vi "SDI_CoordSpace_Test.vi"() -> ()   [LabVIEW 2014]
uses:
  <vilib>/Motion/plugins/PluginFramework/nismSDIFramework.SetFrameworkMode.multi.vi
  <vilib>/Motion/Express/_s/nimc.ex.clearFaults.clearFaults.axis.vi
  <vilib>/Motion/Express/_s/nimc.ex.power.power.axis.vi
  <vilib>/Motion/Express/_s/nimc.ex.straightLineMove.startStraightLineMove.coordinate.modeRelative.0.vi
  <vilib>/Motion/BlockNode/FB.NIMotion.xnode
  <vilib>/Motion/plugins/SDI Plug-in - Delta ASDA/Template SoftMotion Drive Interface Plug-in Class.lvclass
panel:
  in  "Axis 2":refnum<k21>="Axis 2"
  in  "Axis":refnum<k21>="Axis 1"
  in  "velocity":dbl=1000.0
  in  "position[]":dbl[](array[numeric])=[1000.0, 1000.0]
  in  "Coordinate Space":refnum<k21>="SDI Coordinate Space"
  out "error out":errorcluster
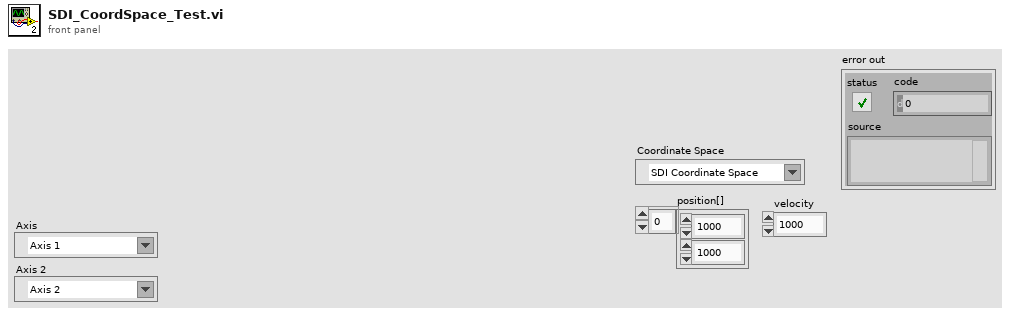
[diagram p1: front panel]
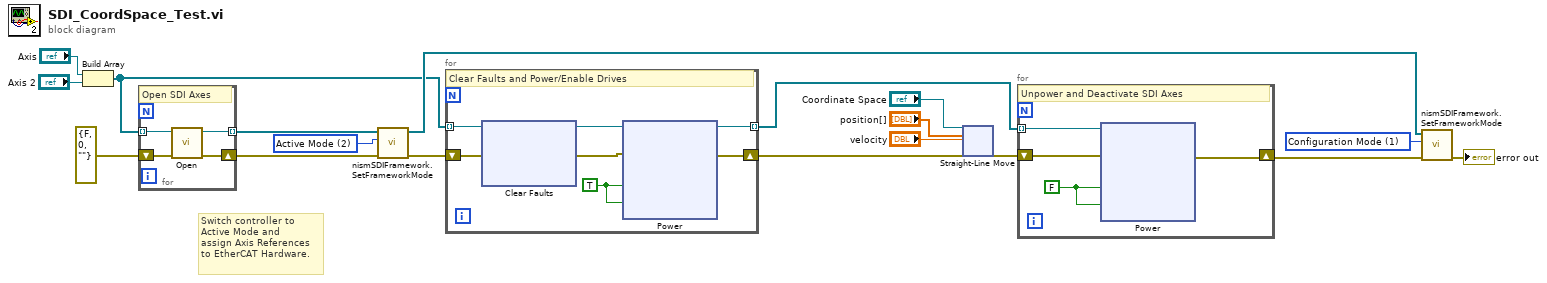
[diagram p0: block diagram]
diagram:
  w13 = 2 items=["Configuration Mode"=1, "Active Mode"=2] ("mode (Active Mode)")
  w16 = 1 items=["Configuration Mode"=1, "Active Mode"=2] ("mode (Active Mode)")
  # "Switch controller to\nActive Mode and \nassign Axis References\nto EtherCAT Hardware."
  n1 = Build Array("Axis", "Axis 2") -> (w7:refnum<k21>[])
  n2 = for {
    tunnel: w7 -> [w22] mode=indexing
    tunnel: [w21] -> w6 mode=indexing
    shift-right: [w20] -> w5
    shift-left: errorcluster {"status"=FALSE, "code"=0, "source"=""} ("error out") -> [w19]
    # "Open SDI Axes"
    n3 = call <vilib>:"Open.vi"("error in (no error)"=w19, "Axis"=w22) -> ("error out"=w20:errorcluster, "Base Axis Out"=w21:refnum<class "nismPluginAxisBaseClass.lvclass">)  [unwired: 8 in]
  }
  n4 = call-poly <vilib>:"nismSDIFramework.SetFrameworkMode.vi"("error in (no error)"=w5, "mode (Active Mode)"=w13, "Base Axis In"=w6) -> ("error out"=w11:errorcluster, "Base Axis Out"=w8:refnum<class "nismPluginAxisBaseClass.lvclass">[])  [unwired: 7 in]
  n5 = for {
    tunnel: w7 -> [w25] mode=indexing
    tunnel: [w24] -> w3 mode=indexing
    shift-right: [w27] -> w9
    shift-left: w11 -> [w26]
    w29 = TRUE ("enable axis")
    # "Clear Faults and Power/Enable Drives"
    n6 = xnode ("Clear Faults")("resource"=w25, "error in"=w26) -> ("resource out"=w23:refnum<k21>, "error out"=w28:errorcluster)
    n7 = xnode ("Power")("enable axis"=w29, "enable drive"=w29, "resource"=w23, "error in"=w28) -> ("resource out"=w24:refnum<k21>, "error out"=w27:errorcluster)
  }
  n8 = xnode ("Straight-Line Move")("resource"="Coordinate Space", "position[]"="position[]", "velocity"="velocity", "error in"=w9) -> ("error out"=w17:errorcluster)  [unwired: 6 in, 2 out]
  n9 = for {
    tunnel: w3 -> [w45] mode=indexing
    shift-right: [w46] -> w15
    shift-left: w17 -> [w44]
    w47 = FALSE ("enable axis")
    # "Unpower and Deactivate SDI Axes"
    n10 = xnode ("Power")("enable axis"=w47, "enable drive"=w47, "resource"=w45, "error in"=w44) -> ("error out"=w46:errorcluster)  [unwired: 1 out]
  }
  n11 = call-poly <vilib>:"nismSDIFramework.SetFrameworkMode.vi"("error in (no error)"=w15, "mode (Active Mode)"=w16, "Base Axis In"=w8) -> ("error out"=→"error out":errorcluster)  [unwired: 7 in, 1 out]
